vi "Open PV Connection.vi"(2 "Error In":errorcluster, 3 "URLs":string[](array[string])) -> (0 "Error Out":errorcluster, 1 "PV Connections":refnum<class "SVConnection.lvclass">[](array[class]))   [LabVIEW 2013, in "CS++ProcessVariables.lvlib" / "SVConnection.lvclass"]
doc: "Opene references to a process variables."
uses:
  SVConnection.lvclass
  PVConnection/PVConnection.lvclass/PVConnection.ctl
  PVConnection/PVConnection.lvclass
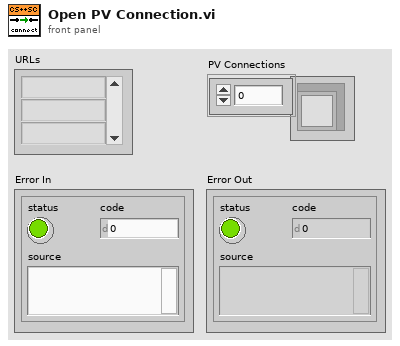
[diagram p1: front panel]
types:
  T1 = cluster{"Write Access":enum8{"Allowed", "Required", "None"}, "Read Access":enum8{"Allowed", "Required", "None"}}
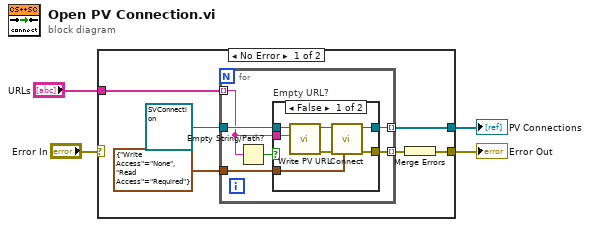
[diagram p0: block diagram]
diagram:
  n1 = case shown="No Error" "Error In" {
    selector: "Error In" -> [_ w25]
    tunnel: "URLs" -> [w8 _]
    tunnel: [w7 _] -> w3
    tunnel: [w5 w25] -> w2
    frame No Error {
      n2 = for {
        tunnel: w8 -> [w12] mode=indexing
        tunnel: refnum<class "SVConnection.lvclass"> refnum ("CS++ProcessVariables.lvlib:SVConnection.lvclass") -> [w16]
        tunnel: T1 {"Write Access"=enum."None", "Read Access"=enum."Required"} ("Access") -> [w15]
        tunnel: [w14] -> w7 mode=indexing
        tunnel: [w11] -> w6 mode=indexing
        n3 = Empty String/Path?(string/path=w12) -> (empty?=w13:bool)
        n4 = case "Empty URL?" shown="False" w13 {
          tunnel: w16 -> [w23 w24]
          tunnel: w12 -> [w22 _]
          tunnel: w15 -> [w19 _]
          tunnel: [w18 w24] -> w14
          tunnel: [w17 _] -> w11
          frame False {
            n5 = call "Write PV URL.vi"("PV URL"=w22, "PVConnection in"=w23) -> ("error out"=w20:errorcluster, "PVConnection out"=w21:refnum<class "SVConnection.lvclass">)  [unwired: 8 in]
            n6 = call-dynamic "Connect.vi"("Access"=w19, "error in (no error)"=w20, "PVConnection in"=w21) -> ("error out"=w17:errorcluster, "PVConnection out"=w18:refnum<class "SVConnection.lvclass">)  [unwired: 7 in]
          }
          frame True {
          }
        }
      }
      n7 = Merge Errors(w6) -> (w5:errorcluster)
    }
    frame Error {
    }
  }
  "PV Connections" <- w3
  "Error Out" <- w2
